vi "all control.vi"() -> (3 "output cluster":T1)   [LabVIEW 2016]
uses:
  Classes/Controller/Motion/A3200 Folder/A3200.lvclass
  Classes/Controller/Dispenser/Ultimus V2 Folder/Ultimus V2.lvclass
  Classes/Controller/I-O/NI-DAQ Folder/NI-DAQ.lvclass
  Classes/Controller/Motion/Motion Folder/Motion.lvclass
  Classes/Controller/I-O/I-O Folder/I-O.lvclass
  Classes/Controller/Dispenser/Dispenser Folder/Dispenser.lvclass
panel:
  in  "Tab Control":T2(tab)
  in  "controller":T3
  in  "IO":cluster{"Output num":dbl[], "Output ":bool[]}
  in  "motion":T4
  in  "dispense":T5={"Vacuum Setting (0000)"=0, "Pressure"=20, "on delay (ms)"=0.5, "off delay (ms) "=0.5} {"Vacuum Setting (0000)" min=0 max=1000 step=1 format="%04.0f"}
  in  "folder and file name":T6={"Path"=path "D:/Gantry_General/Main/ms_kao", "folder name"="data", "file name"="data_", "extension"="txt", "add time string"=FALSE}
  in  "draw point Cluster":T7
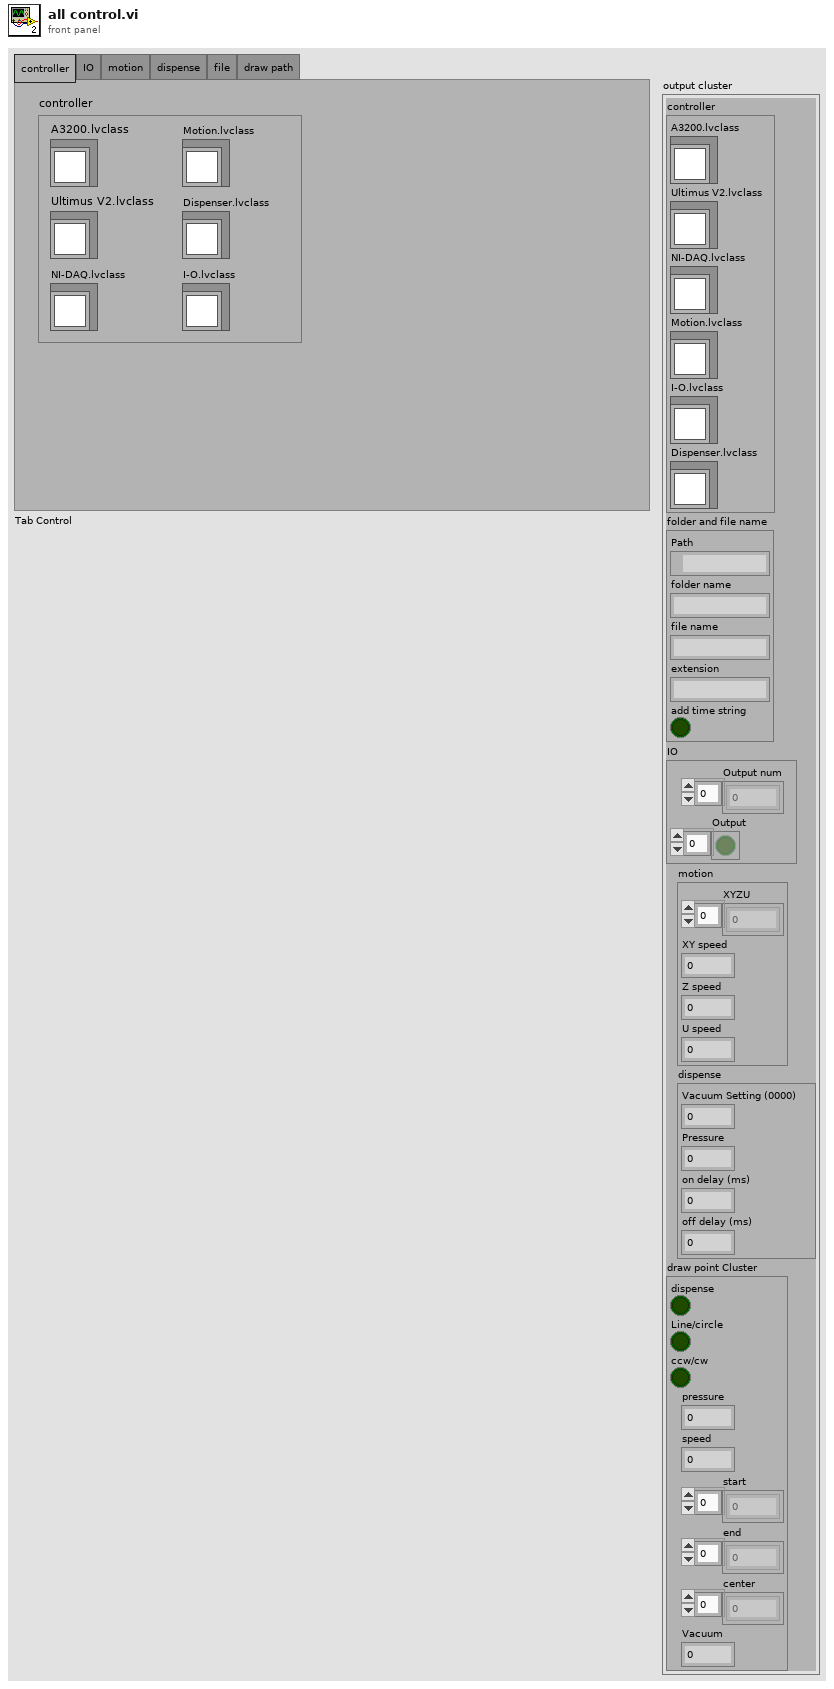
[diagram p1: front panel]
types:
  T1 = cluster{"controller":cluster{"A3200.lvclass":refnum<class "A3200.lvclass">, "Ultimus V2.lvclass":refnum<class "Ultimus V2.lvclass">, "NI-DAQ.lvclass":refnum<class "NI-DAQ.lvclass">, "Motion.lvclass":refnum<class "Motion.lvclass">, "I-O.lvclass":refnum<class "I-O.lvclass">, "Dispenser.lvclass":refnum<class "Dispenser.lvclass">}, "folder and file name":cluster{"Path":path, "folder name":string, "file name":string, "extension":string, "add time string":bool}, "IO":cluster{"Output num":dbl[], "Output ":bool[]}, "motion":cluster{"XYZU ":dbl[], "XY speed":dbl, "Z speed":dbl, "U speed":dbl}, "dispense":cluster{"Vacuum Setting (0000)":i64, "Pressure":i16, "on delay (ms)":dbl, "off delay (ms) ":dbl}, "draw point Cluster":cluster{"dispense":bool, "Line/circle":bool, "ccw/cw":bool, "pressure":dbl, "speed":dbl, "start":dbl[], "end":dbl[], "center":dbl[], "Vacuum":dbl}}
  T2 = enum32{"controller", "IO", "motion", "dispense", "file", "draw path"}
  T3 = cluster{"A3200.lvclass":refnum<class "A3200.lvclass">, "Ultimus V2.lvclass":refnum<class "Ultimus V2.lvclass">, "NI-DAQ.lvclass":refnum<class "NI-DAQ.lvclass">, "Motion.lvclass":refnum<class "Motion.lvclass">, "I-O.lvclass":refnum<class "I-O.lvclass">, "Dispenser.lvclass":refnum<class "Dispenser.lvclass">}
  T4 = cluster{"XYZU ":dbl[], "XY speed":dbl, "Z speed":dbl, "U speed":dbl}
  T5 = cluster{"Vacuum Setting (0000)":i64, "Pressure":i16, "on delay (ms)":dbl, "off delay (ms) ":dbl}
  T6 = cluster{"Path":path, "folder name":string, "file name":string, "extension":string, "add time string":bool}
  T7 = cluster{"dispense":bool, "Line/circle":bool, "ccw/cw":bool, "pressure":dbl, "speed":dbl, "start":dbl[], "end":dbl[], "center":dbl[], "Vacuum":dbl}
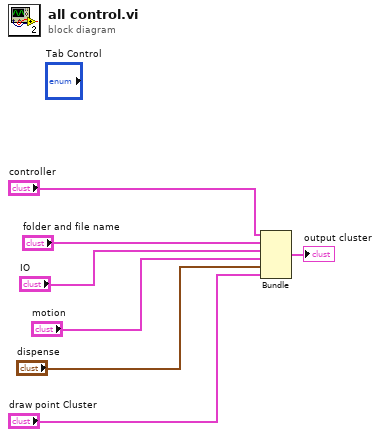
[diagram p0: block diagram]
diagram:
  n1 = Bundle("controller"="controller", "folder and file name"="folder and file name", "IO"="IO", "motion"="motion", "dispense"="dispense", "draw point Cluster"="draw point Cluster") -> (→"output cluster":T1)  [unwired: 1 in]
